vi "PH_DataViewer.get i attribute.vi"(0 "i ref in":refnum<vi>, 5 "error in (no error)":errorcluster) -> (14 "i ref out":refnum<vi>, 16 "i attribute":T1, 19 "error out":errorcluster)   [LabVIEW 2014, in "PH_DataViewer.lvlib"]
doc: "Gets the i attribute data of an object.\n\nLicense Agreement for this software:\n\nCopyright (C)\nGesellschaft für Schwerionenforschung, GSI\nPlanckstr. 1\n64291 Darmstadt\nGermany\n\nContact: D.Beck@gsi.de \n\nThis program is free software; you can redistribute it and/or modify it under the terms of the GNU General Public License as published by the Free Software Foundation; either version 2 of the license, or (at your option) any later version.\n\nThis program is distributed in the hope that it will be useful, but WITHOUT ANY WARRANTY; without even the implied warranty of MERCHANTABILITY or FITNESS FOR A PARTICULAR PURPOSE. See the GNU General License for more details (http://www.gnu.org).\n\nGesellschaft für Schwerionenforschung, GSI\nPlanckstr. 1, 64291 Darmstadt, Germany\nFor all questions and ideas contact: M.Richter@gsi.de, H.Brand@gsi.de or D.Beck@gsi.de.\nLast update: 17-JUN-2004"
uses:
  PH_DataViewer.lvlib
  PH_DataViewer.i attribute.ctl
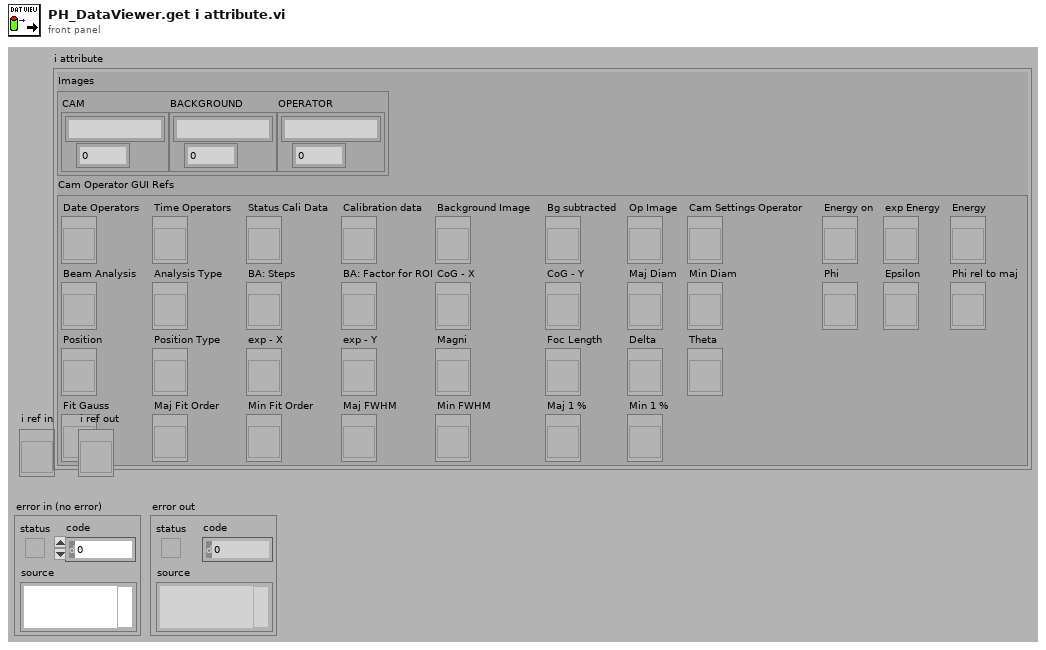
[diagram p1: front panel]
types:
  T1 = typedef "PH_DataViewer.lvlib/PH_DataViewer.i attribute.ctl" = cluster{"Images":cluster{"CAM":cluster{string, u32}, "BACKGROUND":cluster{string, u32}, "OPERATOR":cluster{string, u32}}, "Cam Operator GUI Refs":cluster{"Date Operators":refnum<vi>, "Time Operators":refnum<vi>, "Status Cali Data":refnum<vi>, "Calibration data":refnum<vi>, "Background Image":refnum<vi>, "Bg subtracted":refnum<vi>, "Op Image":refnum<vi>, "Cam Settings Operator":refnum<vi>, "Energy on":refnum<vi>, "exp Energy":refnum<vi>, "Energy":refnum<vi>, "Beam Analysis":refnum<vi>, "Analysis Type":refnum<vi>, "BA: Steps":refnum<vi>, "BA: Factor for ROI":refnum<vi>, "CoG - X":refnum<vi>, "CoG - Y":refnum<vi>, "Maj Diam":refnum<vi>, "Min Diam":refnum<vi>, "Phi":refnum<vi>, "Epsilon":refnum<vi>, "Phi rel to maj":refnum<vi>, "Position":refnum<vi>, "Position Type":refnum<vi>, "exp - X":refnum<vi>, "exp - Y":refnum<vi>, "Magni":refnum<vi>, "Foc Length":refnum<vi>, "Delta":refnum<vi>, "Theta":refnum<vi>, "Fit Gauss":refnum<vi>, "Maj Fit Order":refnum<vi>, "Min Fit Order":refnum<vi>, "Maj FWHM":refnum<vi>, "Min FWHM":refnum<vi>, "Maj 1 %":refnum<vi>, "Min 1 %":refnum<vi>}}
  T2 = enum16{"SetAttribute", "GetAttribute", "CreateAttribute", "DestroyAttribute", "DestroyAllAtributes"}
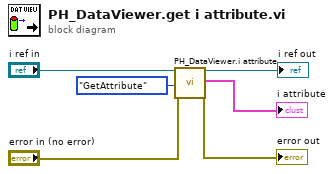
[diagram p0: block diagram]
diagram:
  n1 = call "PH_DataViewer.i attribute.vi"("VI Refnum"="i ref in", "Action"=T2."GetAttribute", "error in (no error)"="error in (no error)") -> ("VI Refnum out"=→"i ref out":refnum<vi>, "CLASS.i attribute out"=→"i attribute":T1, "error out"=→"error out":errorcluster)  [unwired: 14 in]
